vi "模块运行周期接口.vi"(11 "运行周期":T1={"运行模式"=enum."维护模式", "质控频次"=enum."关闭", "空白核查时间"=2, "跨度核查时间"=6, "测量间隔"=240} {"跨度核查时间" items=["00H", "01H", "02H", "03H", "04H", "05H", "06H", "07H", "08H", "09H", "10H", "11H", "12H", "13H", "14H", "15H", "16H", "17H", "18H", "19H", "20H", "21H", "22H", "23H", "关闭"]; "空白核查时间" items=["00H", "01H", "02H", "03H", "04H", "05H", "06H", "07H", "08H", "09H", "10H", "11H", "12H", "13H", "14H", "15H", "16H", "17H", "18H", "19H", "20H", "21H", "22H", "23H", "关闭"]}) -> ()   [LabVIEW 2016]
panel:
  # "运行模式："
  # "质控频次："
  # "零点核查时间："
  # "跨度核查时间："
  # "测量间隔："
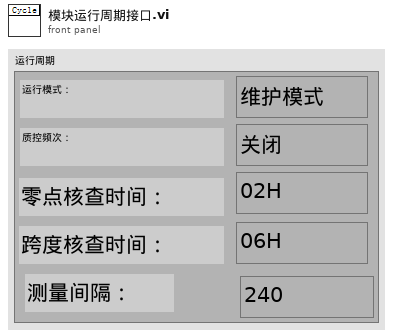
[diagram p1: front panel]
types:
  T1 = cluster{"运行模式":enum16{"维护模式", "常规模式", "应急模式", "质控模式"}, "质控频次":enum16{"关闭", "每天", "星期一", "星期二", "星期三", "星期四", "星期五", "星期六", "星期日"}, "空白核查时间":u16, "跨度核查时间":u16, "测量间隔":u16}
  T2 = cluster{"运行模式":enum16{"维护模式", "常规模式", "应急模式", "质控模式"}, "24H周期设置":bool[]}
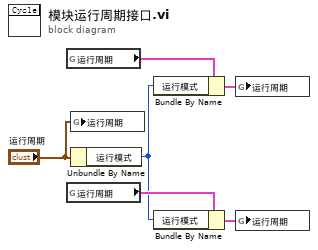
[diagram p0: block diagram]
diagram:
  n1 = global read "断电保存变量.vi" "运行周期"() -> (w6:T2)
  n2 = global read "多参数断电保存全局变量.vi" "运行周期"() -> (w3:T2)
  n3 = global write "总磷总氮断电保存全局变量.vi" "运行周期"("运行周期") -> ()
  n4 = Unbundle By Name("运行周期") -> ("运行模式"=w1:enum16{"维护模式", "常规模式", "应急模式", "质控模式"})
  n5 = Bundle By Name(cluster=w6, "运行模式"=w1) -> (w5:T2)
  n6 = Bundle By Name(cluster=w3, "运行模式"=w1) -> (w2:T2)
  n7 = global write "断电保存变量.vi" "运行周期"(w5) -> ()
  n8 = global write "多参数断电保存全局变量.vi" "运行周期"(w2) -> ()
